vi "ChirpOOPV2.vi"() -> ()   [LabVIEW 2014, in "ChirpV2.lvclass"]
uses:
  ChirpV2.lvclass
  StateV2.ctl
panel:
  out "Stable":bool
  out "#left":i32
  out "?":dbl(slide) scale=0.0..1.0
  out "size(s)":i32
  out "Experiment Variables":T2={"DC_Bias"=0.0, "StartFreq"=0.0, "Duration"=0.0, "State"=enum."Initialization", "window ratio"=0.0, "Final Freq"=0.0}
  out "output cluster":T2={"DC_Bias"=0.0, "StartFreq"=0.0, "Duration"=0.0, "State"=enum."Initialization", "window ratio"=0.0, "Final Freq"=0.0}
  in  "R external(Ohm)":dbl=33.0
  out "error out":errorcluster
  out "Waveform Graph":dynamicdata(graph)
  in  "Path":path=path "C:/Users/YuanYuan/Desktop/Labview Data/Database"
  in  "Sample Name":string="TOKIN1"
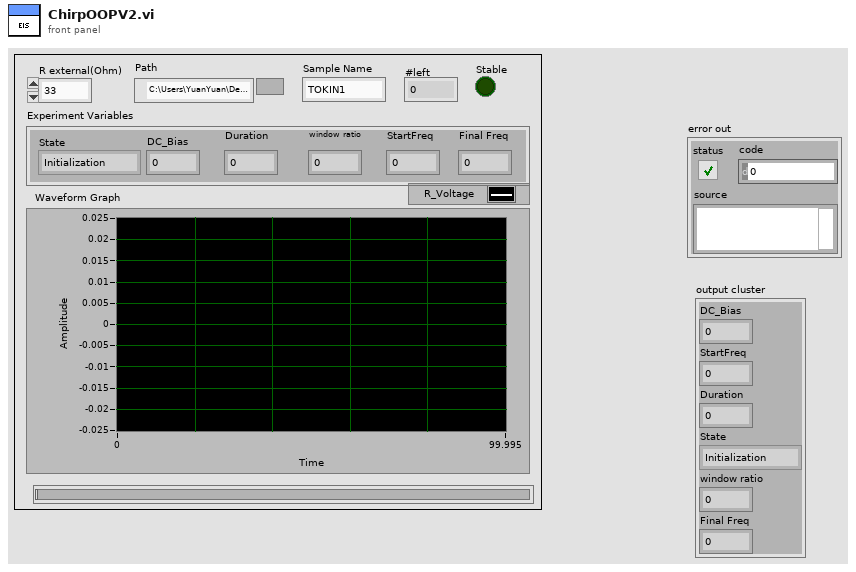
[diagram p1: front panel]
types:
  T1 = typedef "ChirpV2.lvclass/StateV2.ctl" = enum16{"WaitDC", "Initialization", "ChirpSetUp", "Wait", "ChirpMeasurement", "DFT", "WriteData", "Queue", "Ternimation"}
  T2 = cluster{"DC_Bias":dbl, "StartFreq":dbl, "Duration":dbl, "State":T1, "window ratio":dbl, "Final Freq":dbl}
  T3 = cluster{"T":dbl, "Fst":dbl, "Fends":dbl, "Dc":dbl, "w ratio":dbl}
  T4 = cluster{"T":dbl, "Fst":dbl, "Fends":dbl, "Dc":dbl, "w ratio":dbl}[]
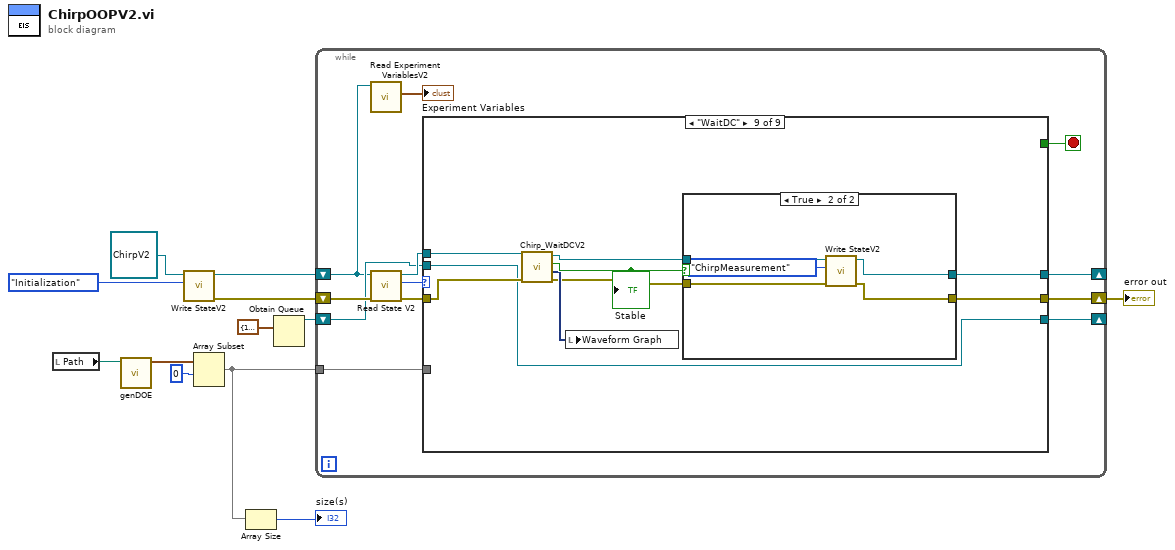
[diagram p0: block diagram]
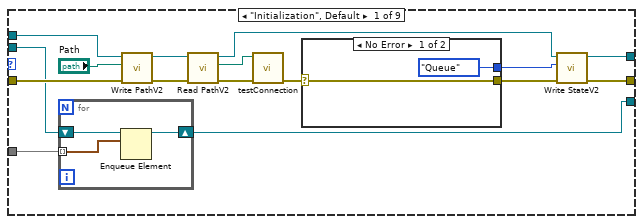
[diagram p2: hidden frame]
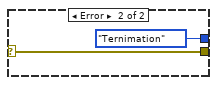
[diagram p3: hidden frame]
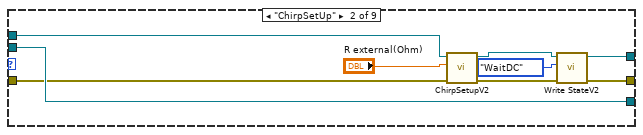
[diagram p4: hidden frame]
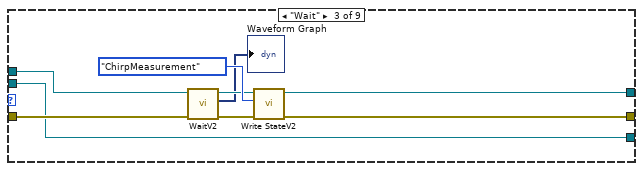
[diagram p5: hidden frame]
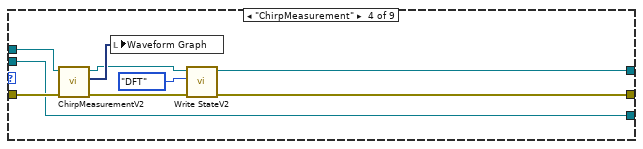
[diagram p6: hidden frame]
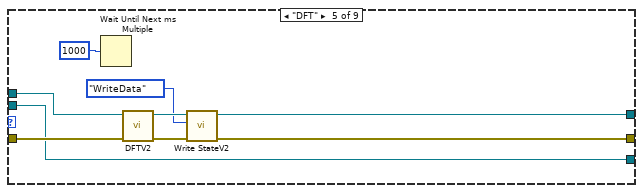
[diagram p7: hidden frame]
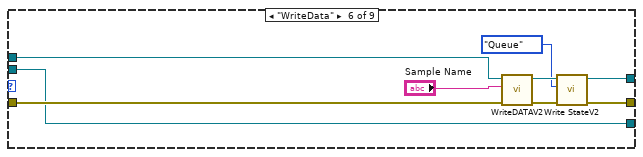
[diagram p8: hidden frame]
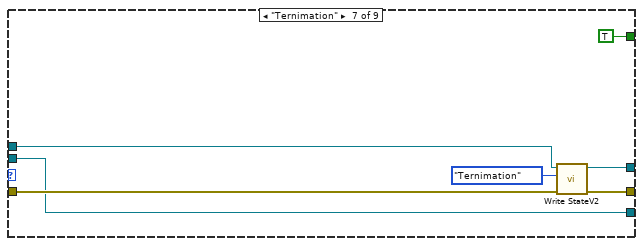
[diagram p9: hidden frame]
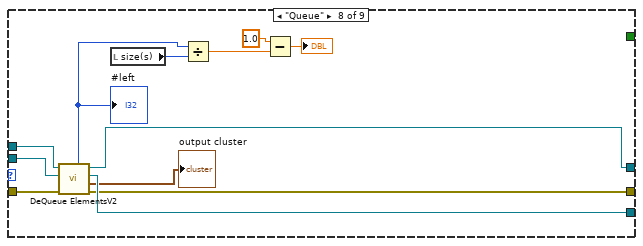
[diagram p10: hidden frame]
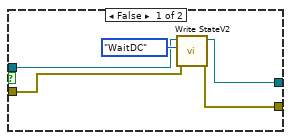
[diagram p11: hidden frame]
diagram:
  n1 = local read "Path"() -> (w5:path)
  n2 = call "genDOE.vi"("db_File"=w5) -> ("Array 2"=w4:T4)  [unwired: 9 in, 1 out]
  n3 = call-dynamic "Write StateV2.vi"("Enum"=StateV2."Initialization", "ChirpV2 in"=refnum<class "ChirpV2.lvclass"> refnum ("ChirpV2.lvclass")) -> ("error out"=w9:errorcluster, "ChirpV2 out"=w10:refnum<class "ChirpV2.lvclass">)  [unwired: 8 in]
  n4 = Array Subset(array=w4, index=0) -> (w3:T4)  [unwired: 1 in]
  n5 = Array Size(array=w3) -> (size(s)=→"size(s)":i32)
  n6 = Obtain Queue(element data type=T3 {"T"=1010.0, "Fst"=0.001, "Fends"=10.0, "Dc"=0.001, "w ratio"=0.001} ("DOE parameters 2")) -> (queue out=w7:refnum<queue>)  [unwired: 4 in, 2 out]
  n7 = while {
    shift-right: [w23] -> _
    shift-left: w10 -> [w14]
    shift-right: [w19] -> w8
    shift-left: w9 -> [w21]
    shift-right: [w16] -> _
    shift-left: w7 -> [w17]
    tunnel: w3 -> [w15]
    stop <- w18 stop-if-true
    n8 = call-dynamic "Read Experiment VariablesV2.vi"("ChirpV2 in"=w14) -> ("Experiment Variables"=→"Experiment Variables":T2)  [unwired: 8 in, 2 out]
    n9 = call-dynamic "Read State V2.vi"("error in (no error)"=w21, "ChirpV2 in"=w14) -> ("error out"=w20:errorcluster, "Enum"=w24:T1, "ChirpV2 out"=w22:refnum<class "ChirpV2.lvclass">)  [unwired: 7 in]
    n10 = case shown="\"WaitDC\"" w24 {
      tunnel: [w39 w53 w61 w71 w77 w87 w98 w107 w115] -> w23
      tunnel: w22 -> [w38 w56 w65 w74 w82 w85 w96 w110 w120]
      tunnel: w20 -> [w37 w48 w64 w73 w81 w92 w95 w109 w119]
      tunnel: [w34 w52 w63 w72 w76 w88 w97 w106 w113] -> w19
      tunnel: [_ _ _ _ _ _ TRUE _ _] -> w18
      tunnel: w17 -> [w27 w50 w57 w66 w75 w84 w93 w111 w112]
      tunnel: [w26 w50 w57 w66 w75 w84 w93 w108 w112] -> w16
      tunnel: w15 -> [w25 _ _ _ _ _ _ _ _]
      frame "Initialization", Default {
        n11 = for {
          shift-right: [w42] -> w26
          shift-left: w27 -> [w43]
          tunnel: w25 -> [w41] mode=indexing
          n12 = Enqueue Element(queue=w43, element=w41) -> (queue out=w42:refnum<queue>)  [unwired: 2 in, 2 out]
        }
        n13 = call-dynamic "Write PathV2.vi"("error in (no error)"=w37, "Path"="Path", "ChirpV2 in"=w38) -> ("error out"=w30:errorcluster, "ChirpV2 out"=w32:refnum<class "ChirpV2.lvclass">)  [unwired: 7 in]
        n14 = call-dynamic "Read PathV2.vi"("error in (no error)"=w30, "ChirpV2 in"=w32) -> ("error out"=w29:errorcluster, "Path"=w28:path, "ChirpV2 out"=w31:refnum<class "ChirpV2.lvclass">)  [unwired: 7 in]
        n15 = call "testConnection.vi"("error in (no error)"=w29, "db_File"=w28) -> ("error out"=w35:errorcluster)  [unwired: 9 in]
        n16 = case shown="No Error" w35 {
          selector: w35 -> [w44 w46]
          tunnel: [StateV2."Queue" ("Enum") StateV2."Ternimation" ("Enum")] -> w40
          tunnel: [w44 w46] -> w33
          frame No Error {
          }
          frame Error {
          }
        }
        n17 = call-dynamic "Write StateV2.vi"("error in (no error)"=w33, "Enum"=w40, "ChirpV2 in"=w31) -> ("error out"=w34:errorcluster, "ChirpV2 out"=w39:refnum<class "ChirpV2.lvclass">)  [unwired: 7 in]
      }
      frame "ChirpSetUp" {
        n18 = call "ChirpSetupV2.vi"("error in (no error)"=w48, "R external(Ohm)"="R external(Ohm)", "ChirpV2 in"=w56) -> ("error out"=w54:errorcluster, "ChirpV2 out"=w55:refnum<class "ChirpV2.lvclass">)  [unwired: 7 in]
        n19 = call-dynamic "Write StateV2.vi"("error in (no error)"=w54, "Enum"=StateV2."WaitDC", "ChirpV2 in"=w55) -> ("error out"=w52:errorcluster, "ChirpV2 out"=w53:refnum<class "ChirpV2.lvclass">)  [unwired: 7 in]
      }
      frame "Wait" {
        n20 = call "WaitV2.vi"("error in (no error)"=w64, "ChirpV2 in"=w65) -> ("error out"=w59:errorcluster, "data"=→"Waveform Graph":dynamicdata, "ChirpV2 out"=w60:refnum<class "ChirpV2.lvclass">)  [unwired: 7 in]
        n21 = call-dynamic "Write StateV2.vi"("error in (no error)"=w59, "Enum"=StateV2."ChirpMeasurement", "ChirpV2 in"=w60) -> ("error out"=w63:errorcluster, "ChirpV2 out"=w61:refnum<class "ChirpV2.lvclass">)  [unwired: 7 in]
      }
      frame "ChirpMeasurement" {
        n22 = call "ChirpMeasurementV2.vi"("error in (no error)"=w73, "ChirpV2 in"=w74) -> ("error out"=w67:errorcluster, "data 3"=w69:dynamicdata, "ChirpV2 out"=w68:refnum<class "ChirpV2.lvclass">)  [unwired: 6 in, 1 out]
        n23 = local write "Waveform Graph"(w69) -> ()
        n24 = call-dynamic "Write StateV2.vi"("error in (no error)"=w67, "Enum"=StateV2."DFT", "ChirpV2 in"=w68) -> ("error out"=w72:errorcluster, "ChirpV2 out"=w71:refnum<class "ChirpV2.lvclass">)  [unwired: 7 in]
      }
      frame "DFT" {
        n25 = Wait Until Next ms Multiple(millisecond multiple=u32 1000) -> ()  [unwired: 1 out]
        n26 = call "DFTV2.vi"("error in (no error)"=w81, "ChirpV2 in"=w82) -> ("error out"=w79:errorcluster, "ChirpV2 out"=w80:refnum<class "ChirpV2.lvclass">)  [unwired: 8 in]
        n27 = call-dynamic "Write StateV2.vi"("error in (no error)"=w79, "Enum"=StateV2."WriteData", "ChirpV2 in"=w80) -> ("error out"=w76:errorcluster, "ChirpV2 out"=w77:refnum<class "ChirpV2.lvclass">)  [unwired: 7 in]
      }
      frame "WriteData" {
        n28 = call "WriteDATAV2.vi"("error in (no error)"=w92, "Sample Name"="Sample Name", "ChirpV2 in"=w85) -> ("error out"=w89:errorcluster, "ChirpV2 out"=w90:refnum<class "ChirpV2.lvclass">)  [unwired: 7 in]
        n29 = call-dynamic "Write StateV2.vi"("error in (no error)"=w89, "Enum"=StateV2."Queue", "ChirpV2 in"=w90) -> ("error out"=w88:errorcluster, "ChirpV2 out"=w87:refnum<class "ChirpV2.lvclass">)  [unwired: 7 in]
      }
      frame "Ternimation" {
        n30 = call-dynamic "Write StateV2.vi"("error in (no error)"=w95, "Enum"=StateV2."Ternimation", "ChirpV2 in"=w96) -> ("error out"=w97:errorcluster, "ChirpV2 out"=w98:refnum<class "ChirpV2.lvclass">)  [unwired: 7 in]
      }
      frame "Queue" {
        n31 = call "DeQueue ElementsV2.vi"("error in (no error)"=w109, "queue in"=w111, "ChirpV2 in"=w110) -> ("error out"=w106:errorcluster, "output cluster"=→"output cluster":T2, "queue out"=w108:refnum<queue>, "ChirpV2 out"=w107:refnum<class "ChirpV2.lvclass">, "#left"=w104:i32)  [unwired: 4 in]
        "#left" <- w104
        n32 = local read "size(s)"() -> (w103:i32)
        n33 = Divide(x=w104, y=w103) -> (x/y=w102:dbl)
        n34 = Subtract(x=1.0, y=w102) -> (x-y=→"?":dbl)
      }
      frame "WaitDC" {
        n35 = call-dynamic "Chirp_WaitDCV2.vi"("error in (no error)"=w119, "ChirpV2 in"=w120) -> ("error IO"=w114:errorcluster, "data"=w116:dynamicdata, "Boolean"=w117:bool, "ChirpV2 out"=w118:refnum<class "ChirpV2.lvclass">)  [unwired: 6 in]
        "Stable" <- w117
        n36 = local write "Waveform Graph"(w116) -> ()
        n37 = case shown="True" w117 {
          tunnel: w118 -> [w124 w130]
          tunnel: [w122 w128] -> w115
          tunnel: w114 -> [w123 w127]
          tunnel: [w121 w126] -> w113
          frame False {
            n38 = call-dynamic "Write StateV2.vi"("error in (no error)"=w123, "Enum"=StateV2."WaitDC", "ChirpV2 in"=w124) -> ("error out"=w121:errorcluster, "ChirpV2 out"=w122:refnum<class "ChirpV2.lvclass">)  [unwired: 7 in]
          }
          frame True {
            n39 = call-dynamic "Write StateV2.vi"("error in (no error)"=w127, "Enum"=StateV2."ChirpMeasurement", "ChirpV2 in"=w130) -> ("error out"=w126:errorcluster, "ChirpV2 out"=w128:refnum<class "ChirpV2.lvclass">)  [unwired: 7 in]
          }
        }
      }
    }
  }
  "error out" <- w8
